vi "download_calibration_rm_imu.vi"(9 "port":u16, 10 "host":string, 11 "path in":path=path "hl2ss_ulm.dll") -> (1 "error":bool, 2 "calibration":cluster{"extrinsics":sgl[][]}, 3 "path out":path)   [LabVIEW 2023]
panel:
  in  "calibration":cluster{"extrinsics":sgl[][]}
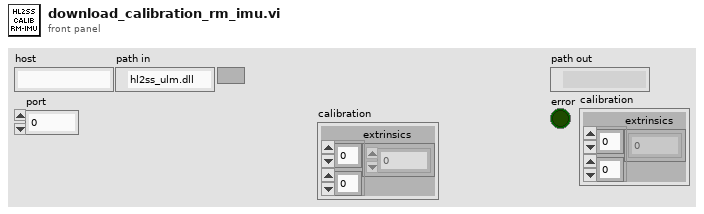
[diagram p1: front panel]
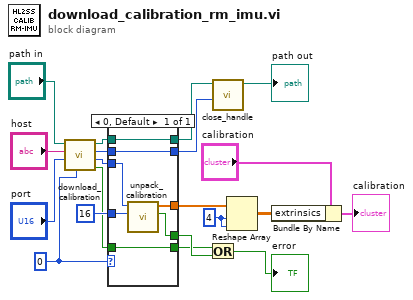
[diagram p0: block diagram]
diagram:
  w8 = 4 ("dimension size")
  w17 = u64 0 ("configuration")
  n1 = call "download_calibration.vi"("configuration"=w17, "port"="port", "host"="host", "path in"="path in") -> ("error"=w5:bool, "calibration"=w15:u64, "calibration_handle"=w13:u64, "path out"=w14:path)  [unwired: 4 in]
  n2 = case shown="0, Default" w17 {
    tunnel: 16 ("element_count") -> [w27]
    tunnel: w15 -> [w26]
    tunnel: w14 -> [w25]
    tunnel: w13 -> [w24]
    tunnel: [w25] -> w12
    tunnel: [w24] -> w11
    tunnel: [w23] -> w4
    tunnel: [w22] -> w10
    tunnel: [w21] -> w6
    tunnel: w5 -> [w21]
    frame 0, Default {
      n3 = call "unpack_calibration.vi"("element_count"=w27, "calibration"=w26) -> ("error"=w22:bool, "calibration"=w23:sgl[])  [unwired: 8 in]
    }
  }
  n4 = Or(x=w6, y=w10) -> (x .or. y?=→"error":bool)
  n5 = call "close_handle.vi"("handle"=w11, "path in"=w12) -> ("path out"=→"path out":path)  [unwired: 9 in]
  n6 = Reshape Array(w4, w8, w8) -> (w2:sgl[][])
  n7 = Bundle By Name(cluster="calibration", "extrinsics"=w2) -> (→"calibration":cluster{"extrinsics":sgl[][]})
